vi "Open.vi"(8 "error in (no error)":errorcluster, 10 "address":string, 11 "instrument.Cryostation in":refnum<class "instrument.Cryostation.lvclass">) -> (0 "error out":errorcluster, 3 "instrument.Cryostation out":refnum<class "instrument.Cryostation.lvclass">)   [LabVIEW 2019, in "instrument.Cryostation.lvclass"]
uses:
  instrument.Cryostation.lvclass
  C:/Program Files (x86)/National Instruments/LabVIEW 2019/user.lib/LevyLab/Levylab Instruments/SMOs/Instrument/Instrument.lvclass
  <userlib>/LevyLab/Instrument Framework/Instrument Types/Cryostat/Instrument.Cryostat.lvclass
  <userlib>/LevyLab/Instrument Framework/SMOs/Instrument/Instrument.lvclass
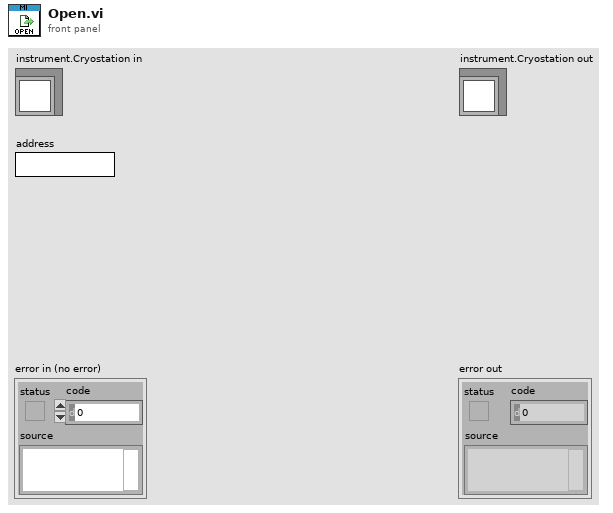
[diagram p1: front panel]
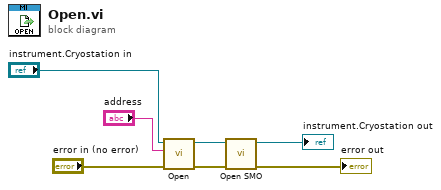
[diagram p0: block diagram]
diagram:
  n1 = call-parent "Open.vi"("error in (no error)"="error in (no error)", "address"="address", "Instrument in"="instrument.Cryostation in") -> ("error out"=w3:errorcluster, "Instrument out"=w4:refnum<class "instrument.Cryostation.lvclass">)  [unwired: 7 in]
  n2 = call <userlib>:"Open SMO.vi"("error in (no error)"=w3, "Instrument in"=w4) -> ("error out"=→"error out":errorcluster, "Instrument out"=→"instrument.Cryostation out":refnum<class "instrument.Cryostation.lvclass">)  [unwired: 8 in]
